vi "Protocol.Close References.vi"(8 "error in":errorcluster, 11 "J1939 Cluster":T1) -> (0 "error out":errorcluster)   [LabVIEW 2019, in "J1939 Addon Engine.lvlib"]
uses:
  J1939 Addon Engine.lvlib
  Types/Protocol.Refs.ctl
  Shared/J1939 Utilities/Types/CAN Outgoing Message Cluster.ctl
  Types/Protocol.RQST Lookup Table Reference.ctl
  Types/Protocol.Address Table Reference.ctl
  Shared/J1939 Utilities/J1939 Utilities.lvlib
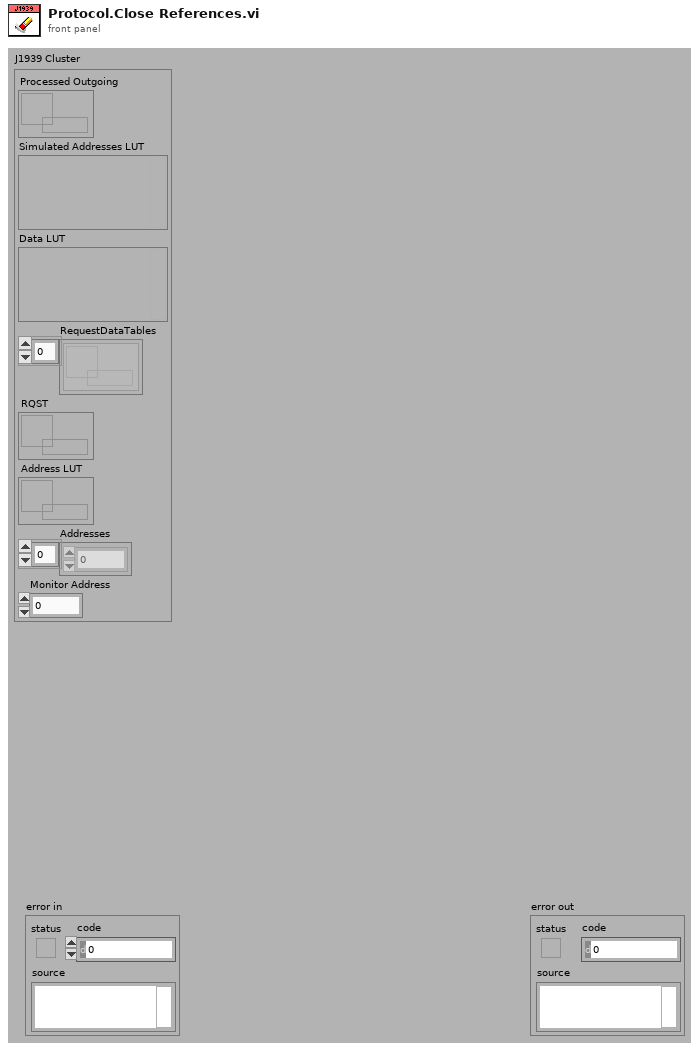
[diagram p1: front panel]
types:
  T1 = typedef "J1939 Addon Engine.lvlib/Protocol.Refs.ctl" = cluster{"Processed Outgoing":refnum<queue>, "Simulated Addresses LUT":variant, "Data LUT":variant, "RequestDataTables":refnum<k33>[], "RQST":T2, "Address LUT":T3, "Addresses":u8[], "Monitor Address":u8}
  T2 = typedef "J1939 Addon Engine.lvlib/Protocol.RQST Lookup Table Reference.ctl" = refnum<data-value>
  T3 = typedef "J1939 Addon Engine.lvlib/Protocol.Address Table Reference.ctl" = refnum<data-value>
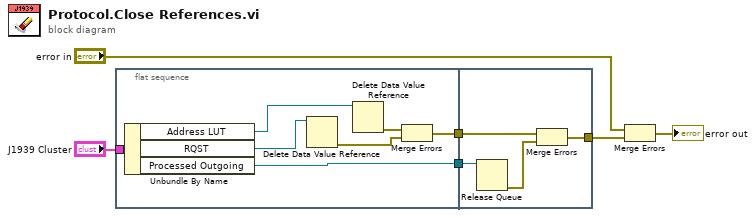
[diagram p0: block diagram]
diagram:
  n1 = flat-sequence {
    tunnel: "J1939 Cluster" -> [w10]
    tunnel: [w11] -> w5
    tunnel: [w9] -> w1
    tunnel: w5 -> [w17]
    tunnel: [w15] -> w4
    tunnel: w1 -> [w14]
    frame #0 {
      n2 = Unbundle By Name(w10) -> ("Address LUT"=w7:T3, "RQST"=w8:T2, "Processed Outgoing"=w9:refnum<queue>)
      n3 = Delete Data Value Reference(data value reference=w8) -> (error out=w12:errorcluster)  [unwired: 1 in, 1 out]
      n4 = Delete Data Value Reference(data value reference=w7) -> (error out=w13:errorcluster)  [unwired: 1 in, 1 out]
      n5 = Merge Errors(w13, w12) -> (w11:errorcluster)
    }
    frame #1 {
      n6 = Release Queue(queue=w14) -> (error out=w16:errorcluster)  [unwired: 2 in, 2 out]
      n7 = Merge Errors(w17, w16) -> (w15:errorcluster)
    }
  }
  n8 = Merge Errors("error in", w4) -> (→"error out":errorcluster)
